vi "GE 5565PIORC.Registers.Local Configuration.Read (U8).vi"(7 "Mask (0xFF)":u8=255 format="%.0x", 8 "error in (no error)":errorcluster, 10 "Register":T1=8 items=["MARBR"=8, "BIGEND"=12, "INTCSR"=104, "PCIHREV"=116, "DMAMODE0"=128, "DMAPADR0"=132, "DMALADR0"=136, "DMASIZ0"=140, "DMADPR0"=144, "DMACSR0"=168, "DMADAC0"=180, "LAS1RR"=240, "LAS1BA"=244], 11 "GE 5565PIORC in":refnum<class "GE 5565PIORC.lvclass">) -> (0 "error out":errorcluster, 1 "Value":u8, 3 "GE 5565PIORC out":refnum<class "GE 5565PIORC.lvclass">)   [LabVIEW 2020, in "GE 5565PIORC.lvclass"]
uses:
  GE 5565PIORC.lvclass
  GE 5565PIORC.Registers.Local Configuration.ctl
  <vilib>/Instr/_visa.llb/VISA Register Access Address Space.ctl
  GE 5565PIORC.lvclass/GE 5565PIORC.ctl
  Methods/GE 5565PIORC.Registers.Read (U8).vi
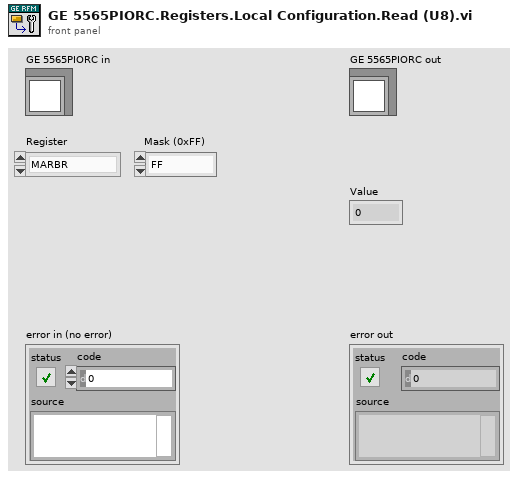
[diagram p1: front panel]
types:
  T1 = typedef "GE 5565PIORC.lvclass/GE 5565PIORC.Registers.Local Configuration.ctl" = u32
  T2 = typedef "VISA Register Access Address Space.ctl" = u16
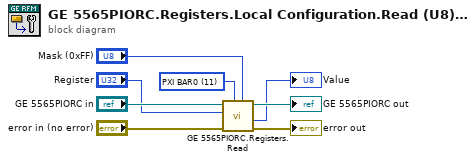
[diagram p0: block diagram]
diagram:
  w4 = T2 11 items=["VXI/VME A16"=1, "VXI/VME A24"=2, "VXI/VME A32"=3, "VXI/VME A64"=4, "PXI Memory Allocations"=9, "PXI Configuration"=10, "PXI BAR0"=11, "PXI BAR1"=12, "PXI BAR2"=13, "PXI BAR3"=14, "PXI BAR4"=15, "PXI BAR5"=16] ("Address Space")
  n1 = call-poly "GE 5565PIORC.Registers.Read.vi"("Mask (0xFF)"="Mask (0xFF)", "Address Space"=w4, "error in (no error)"="error in (no error)", "Offset"="Register", "GE 5565PIORC in"="GE 5565PIORC in") -> ("error out"=→"error out":errorcluster, "Value"=→"Value":u8, "GE 5565PIORC out"=→"GE 5565PIORC out":refnum<class "GE 5565PIORC.lvclass">)  [unwired: 4 in]
